vi "Test - Extract_multipart_message.vi"() -> ()   [LabVIEW 2019, in "mmW_commands.lvlib"]
uses:
  mmW_commands.lvlib
  TypeDefs/commands.ctl
panel:
  out "Evaluation":T2(array[cluster])
  out "last message":string[](array[string])
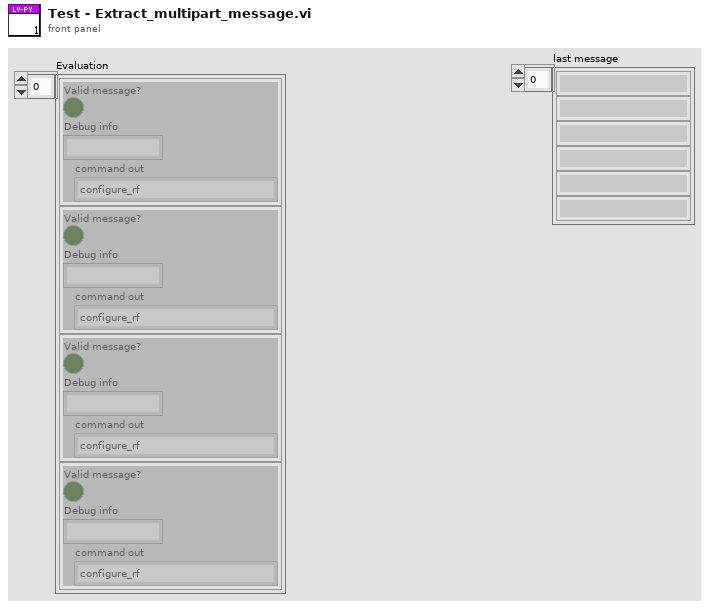
[diagram p1: front panel]
types:
  T1 = typedef "mmW_commands.lvlib/commands.ctl" = enum16{"configure_fs", "configure_rf", "configure_trigger", "equalization_enable", "equalization_start", "lo_sync_enable", "equalization_stop", "get_instrument_status", "get_versions", "initialize_hw", "pop_rx", "set_log_level", "Shutdown", "start", "start_instrument_app", "stop", "trans", "transceive", "trigger_burst", "trigger_sync_enable", "Write TX", "resp_generic", "resp_waveform", "send_trigger", "fetch", "transceive2"}
  T2 = cluster{"Valid message?":bool, "Debug info":string, "command out":T1}[]
  T3 = typedef "mmW_commands.lvlib/commands_instrument_control.ctl" = enum16{"configure_rf", "configure_rx_sync", "configure_trigger", "initialize_hw", "pop_rx", "set_mode", "shutdown", "start", "stop", "trigger_burst", "write_tx"}
  T4 = cluster{"Valid message?":bool, "Debug info":string, "command out":T3}
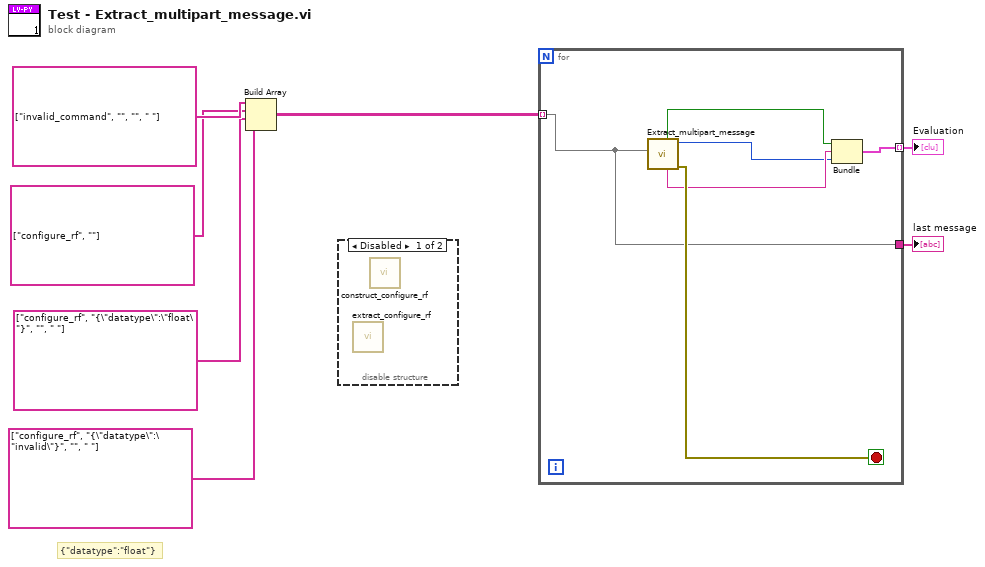
[diagram p0: block diagram]
diagram:
  # "{\"datatype\":\"float\"}"
  n1 = Build Array(string[] ["invalid_command", "", "", " "] ("multipart message in"), string[] ["configure_rf", ""] ("multipart message in"), string[] ["configure_rf", "{\"datatype\":\"float\"}", "", " "] ("multipart message in"), string[] ["configure_rf", "{\"datatype\":\"invalid\"}", "", " "] ("multipart message in")) -> (w3:string[][])
  n2 = disable-structure shown="Disabled" {
    frame Disabled {
      n3 = call "extract_configure_rf.vi"() -> ()  [unwired: 10 in, 6 out]
      n4 = call "construct_configure_rf.vi"() -> ()  [unwired: 11 in, 5 out]
    }
    frame Enabled {
    }
  }
  n5 = for {
    tunnel: w3 -> [w12] mode=indexing
    tunnel: [w12] -> w2
    tunnel: [w9] -> w1 mode=indexing
    stop <- w13 stop-if-true
    n6 = call "Extract_multipart_message.vi"("multipart message in"=w12) -> ("error out"=w13:errorcluster, "command out"=w8:T3, "Debug info"=w10:string, "Valid message?"=w11:bool)  [unwired: 5 in, 2 out]
    n7 = Bundle("Valid message?"=w11, "Debug info"=w10, "command out"=w8) -> (w9:T4)  [unwired: 1 in]
  }
  "last message" <- w2
  "Evaluation" <- w1
